vi "Get Timestamp Filename String.vi"() -> (0 "time format string":string)   [LabVIEW 2021, in "Logging.lvlib"]
doc: "Get the format string for specifying a timestamp that can be used as part of a file name."
uses:
  Logging.lvlib
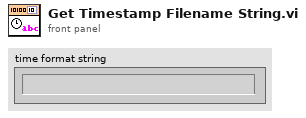
[diagram p1: front panel]
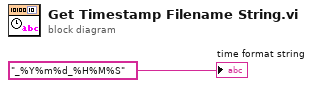
[diagram p0: block diagram]
diagram:
  "time format string" <- "_%Y%m%d_%H%M%S" ("time format string (%c)")
